vi "ModifyAttribute2.vi"(0 "reference in":refnum<class "G#SubSubClass2.lvclass">, 1 "Lock time (ms)":u32, 2 "timeout in ms (-1)":i32=-1, 3 "Unlock data if error? (T)":bool=TRUE, 4 "Only unlock data? (F)":bool, 5 "error in (no error)":errorcluster) -> (14 "reference out":refnum<class "G#SubSubClass2.lvclass">, 16 "timeout":bool, 19 "error out":errorcluster)   [LabVIEW 2010, in "G#SubSubClass2.lvclass"]
uses:
  G#SubSubClass2.lvclass
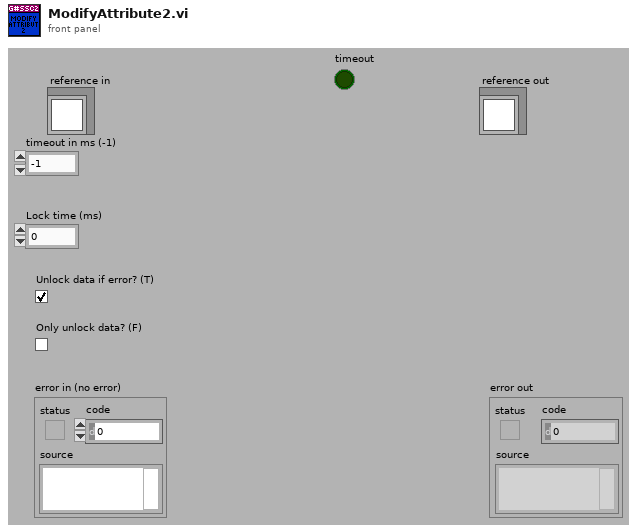
[diagram p1: front panel]
types:
  T1 = typedef "G#SubSubClass2.lvclass/ObjectAttributes.ctl" = cluster{"Base class":T2, "SubSubAttribute":dbl}
  T2 = typedef "G#SubClass2.lvclass/ObjectAttributes.ctl" = cluster{"Base class":T3, "SubAttribute":dbl}
  T3 = typedef "G#BaseClass2.lvclass/ObjectAttributes.ctl" = cluster{"Numeric":dbl, "Array":dbl[]}
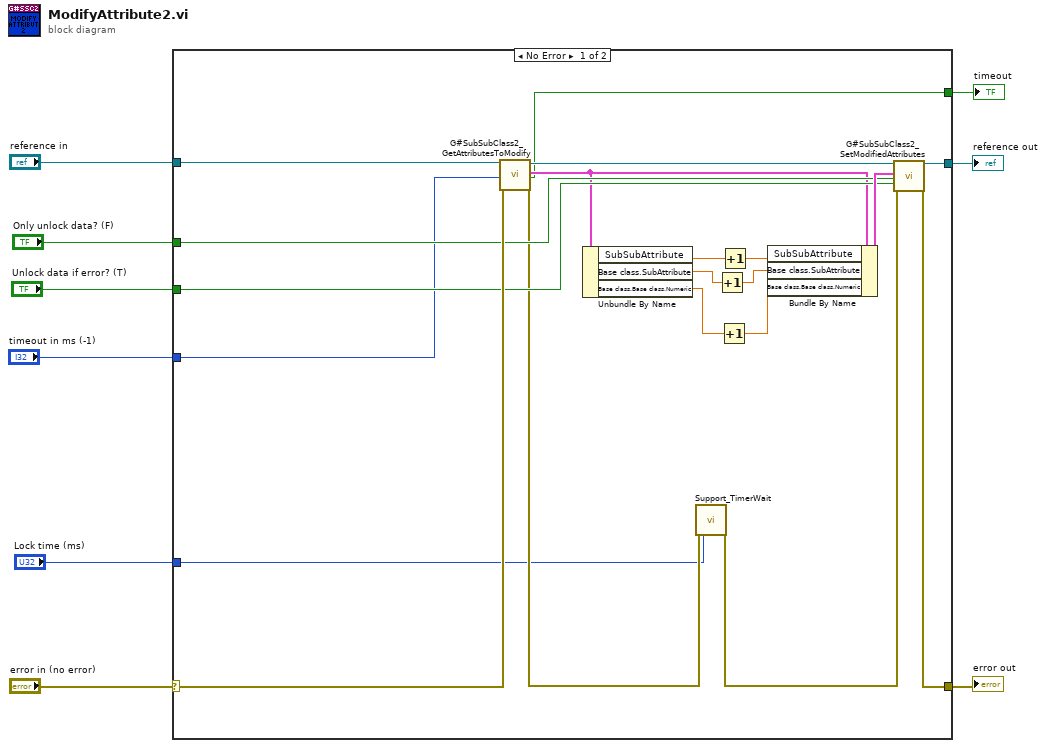
[diagram p0: block diagram]
diagram:
  n1 = case shown="No Error" "error in (no error)" {
    selector: "error in (no error)" -> [w25 w31]
    tunnel: [w27 w31] -> w8
    tunnel: [w24 w30] -> w6
    tunnel: "reference in" -> [w26 w30]
    tunnel: "Only unlock data? (F)" -> [w23 _]
    tunnel: "Unlock data if error? (T)" -> [w22 _]
    tunnel: "Lock time (ms)" -> [w12 _]
    tunnel: [w11 _] -> w2
    tunnel: "timeout in ms (-1)" -> [w10 _]
    frame No Error {
      n2 = call "G#SubSubClass2_GetAttributesToModify.vi"("reference in"=w26, "timeout in ms (-1)"=w10, "error in (no error)"=w25) -> ("reference out"=w28:refnum<class "G#SubSubClass2.lvclass">, "attributes"=w21:T1, "timeout"=w11:bool, "error out"=w14:errorcluster)  [unwired: 12 in, 1 out]
      n3 = Unbundle By Name(w21) -> ("SubSubAttribute"=w20:dbl, "Base class.SubAttribute"=w18:dbl, "Base class.Base class.Numeric"=w16:dbl)
      n4 = call "Support_TimerWait.vi"("error in (no error)"=w14, "milliseconds to wait"=w12) -> ("error out"=w13:errorcluster)  [unwired: 17 in]
      n5 = Increment(x=w18) -> (x+1=w17:dbl)
      n6 = Increment(x=w16) -> (x+1=w15:dbl)
      n7 = Increment(x=w20) -> (x+1=w19:dbl)
      n8 = Bundle By Name(cluster=w21, "SubSubAttribute"=w19, "Base class.SubAttribute"=w17, "Base class.Base class.Numeric"=w15) -> (w29:T1)
      n9 = call "G#SubSubClass2_SetModifiedAttributes.vi"("reference in"=w28, "attributes"=w29, "Only unlock data? (F)"=w23, "Unlock data if error? (T)"=w22, "error in (no error)"=w13) -> ("reference out"=w24:refnum<class "G#SubSubClass2.lvclass">, "error out"=w27:errorcluster)  [unwired: 13 in]
    }
    frame Error {
    }
  }
  "error out" <- w8
  "reference out" <- w6
  "timeout" <- w2
